vi "Actor Core.vi"(8 "error in":errorcluster, 11 "Nested in":refnum<class "UI Actor.lvclass">) -> (0 "error out":errorcluster, 3 "Actor out":refnum<class "Actor.lvclass">)   [LabVIEW 2019, in "UI Actor.lvlib" / "UI Actor.lvclass"]
doc: "(<B>Filename</B>: Actor Framework.lvlib:Actor.lvclass:Actor Core.vi)\n\nReceives messages to the actor, reacts to them, and initiates any error handling that may shut the actor down.\n\nDescendant classes may override this VI to append parallel tasks for the actor to complete while it handles messages. Overrides use the Call Parent Method node."
uses:
  UI Actor.lvclass
  C:/Program Files (x86)/National Instruments/LabVIEW 2019/vi.lib/ActorFramework/Actor/Actor.lvclass
  <vilib>/ActorFramework/Actor/Actor.lvclass
  UI Actor.lvclass/UI Actor.ctl
  <vilib>/ActorFramework/Actor/Actor.lvclass/Actor.ctl
  <vilib>/ActorFramework/Message Enqueuer/Message Enqueuer.lvclass/Message Enqueuer.ctl
  Write Sub Panel Monedas.vi
  Write Sub Panel Productos.vi
  Write Sub Panel Msg.vi
  <vilib>/ActorFramework/Message Enqueuer/Init from Existing Queue.vi
  <vilib>/ActorFramework/Message Enqueuer/Enqueue.vi
  <vilib>/ActorFramework/Stop Msg/Stop Msg.lvclass
  C:/Program Files (x86)/National Instruments/LabVIEW 2019/vi.lib/ActorFramework/Message/Message.lvclass
  <vilib>/ActorFramework/Message Priority Queue/Priority Enqueue.vi
  <vilib>/ActorFramework/Message Enqueuer/Message Enqueuer.lvclass
panel:
  out "PRODUCTO COMPRADO":T1
  out "CREDITO":dbl
  out "PRODUCTO SELECCIONADO":string
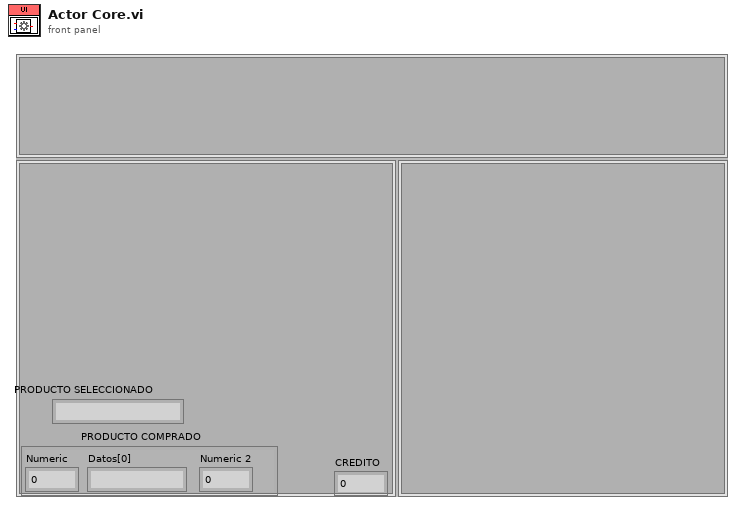
[diagram p1: front panel]
types:
  T1 = cluster{"Numeric":i32, "Datos[0]":string, "Numeric 2":dbl}
  T2 = cluster{"Stop":refnum<user-event>, "CREDITO":refnum<user-event>, "PRODUCTO COMPRADO":refnum<user-event>, "PRODUCTO SELECCIONADO":refnum<user-event>}
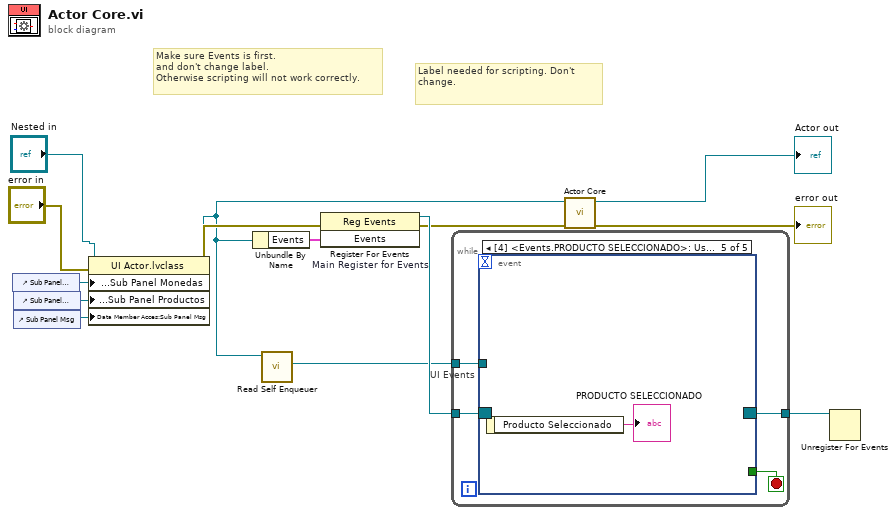
[diagram p0: block diagram]
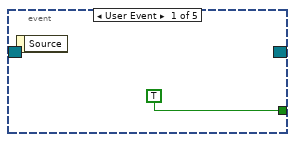
[diagram p2: hidden frame]
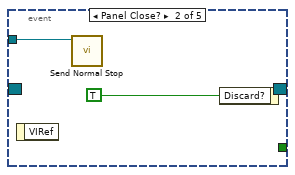
[diagram p3: hidden frame]
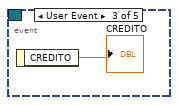
[diagram p4: hidden frame]
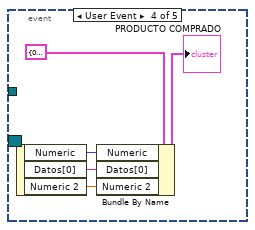
[diagram p5: hidden frame]
diagram:
  # "Label needed for scripting. Don't change."
  # "Make sure Events is first.\nand don't change label.\nOtherwise scripting will not work correctly."
  n1 = control-ref of="Sub Panel Monedas"() -> (w4:refnum<vi>)
  n2 = control-ref of="Sub Panel Productos"() -> (w3:refnum<vi>)
  n3 = control-ref of="Sub Panel Msg"() -> (w2:refnum<vi>)
  n4 = property class="UI Actor.lvclass"(reference="Nested in", error in="error in", "Data Member Acces:Sub Panel Monedas"=w4, "Data Member Acces:Sub Panel Productos"=w3, "Data Member Acces:Sub Panel Msg"=w2) -> (reference out=w5:refnum<class "UI Actor.lvclass">, error out=w7:errorcluster)
  n5 = Unbundle By Name(w5) -> ("Events"=w11:T2)
  n6 = call <vilib>:"Read Self Enqueuer.vi"("Actor"=w5) -> ("Self Enqueuer"=w9:refnum<class "Message Enqueuer.lvclass">)  [unwired: 10 in]
  n7 = register-events "Main Register for Events"(error in=w7, w11) -> (reference out=w12:refnum<event-registration>, error out=w8:errorcluster)  [unwired: 1 in]
  n8 = while {
    tunnel: w12 -> [w18]
    tunnel: [w16] -> w10
    tunnel: w9 -> [w15]
    stop <- w17 stop-if-true
    n9 = event "UI Events" shown="[4] <Events.PRODUCTO SELECCIONADO>: User Event" {
      selector: w18 -> [_ _ _ _ _]
      dyn-events: [_ _ _ _ _] -> w16
      timeout: _ -> [_ _ _ _ _]
      tunnel: [TRUE _ _ _ _] -> w17
      tunnel: w15 -> [_ w20 _ _ _]
      event User Event {
        n10 = event-data() -> ()  [unwired: 1 in, 1 out]
      }
      event Panel Close? {
        n11 = event-data() -> ()  [unwired: 1 in, 1 out]
        n12 = call <vilib>:"Send Normal Stop.vi"("Message Enqueuer"=w20) -> ()  [unwired: 10 in, 1 out]
        n13 = event-data("Discard?"=TRUE) -> ()  [unwired: 1 in, 1 out]
      }
      event User Event {
        n14 = event-data() -> ("CREDITO"=→"CREDITO":dbl)  [unwired: 1 in]
      }
      event User Event {
        n15 = event-data() -> ("Numeric"=w26:i32, "Datos[0]"=w25:string, "Numeric 2"=w24:dbl)  [unwired: 1 in]
        n16 = Bundle By Name(cluster=T1 {"Numeric"=0, "Datos[0]"="", "Numeric 2"=0.0} ("PRODUCTOS"), "Numeric"=w26, "Datos[0]"=w25, "Numeric 2"=w24) -> (→"PRODUCTO COMPRADO":T1)
      }
      event User Event {
        n17 = event-data() -> ("Producto Seleccionado"=→"PRODUCTO SELECCIONADO":string)  [unwired: 1 in]
      }
    }
  }
  n18 = call-parent "Actor Core.vi"("error in"=w8, "Actor in"=w5) -> ("error out"=→"error out":errorcluster, "Actor out"=→"Actor out":refnum<class "Actor.lvclass">)  [unwired: 8 in]
  n19 = Unregister For Events(event registration refnum=w10) -> ()  [unwired: 1 in, 1 out]
